vi "_test_BC_FromScratch.vi"() -> ()   [LabVIEW 2020]
uses:
  Source/Libraries/Ballard_1553_Hardware_ni/_typedefs/MessageBuffer_type.ctl
  Source/Libraries/Ballard_1553_Hardware_ni/_typedefs/MessageCommand_BCRT_type.ctl
  <vilib>/addons/_JKI Toolkits/Caraya/classes/Assert/Assert Not Error.vi
  <vilib>/addons/_JKI Toolkits/Caraya/classes/Assert/Assert.lvclass
  <vilib>/addons/_JKI Toolkits/Caraya/classes/Test/Test.lvclass
  Source/Libraries/Ballard_1553_Hardware_ni/Ballard_1553_Hardware_ni.lvlib
panel:
  in  "bus monitor":string="busMonitor"
  in  "major frame":string="testMajorFrame"
  in  "minor frame":string="testMinorFrame"
  in  "message command name":string="testBCmsg"
  in  "message buffer name":string="testBCmsgBuffer"
  in  "BC name":string="testBC"
  in  "channel name":string="channel1553"
  in  "Message Command Configuration":T1={"taVal1"=1, "saVal1"=2, "wordCount1"=1}
  in  "MessageBuffer configuration":T2={"bufferMaxEntries"=1, "bufferType"=0, "eventLogOnEmptyOrFull"=FALSE, "eventLogOnHalf"=FALSE} {"bufferType" items=["FIFO", "Circular"]}
  in  "XML Configuration File Path":path=path "C:/Users/Administrator/Desktop/GIT/Ballard-Arinc-429-XML-Generator/Database Examples/HardwareBallard_1553_Scripted.xml"
  out "error out":errorcluster
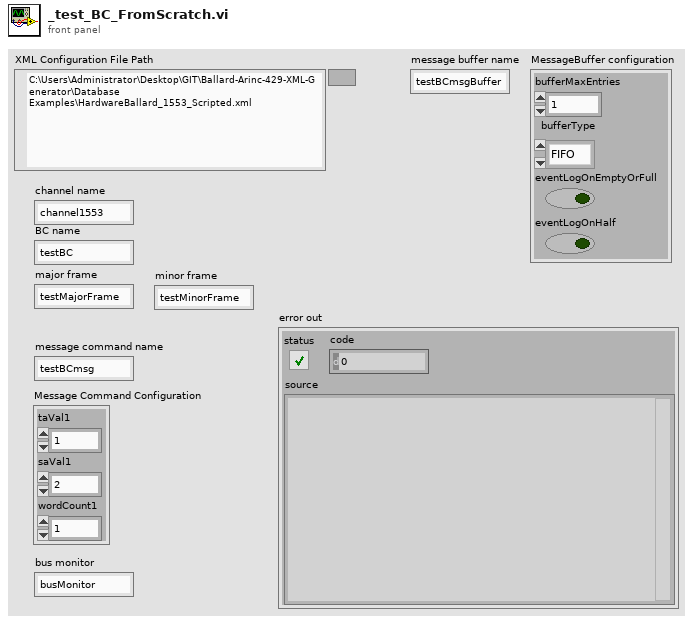
[diagram p1: front panel]
types:
  T1 = typedef "Ballard_1553_Hardware_ni.lvlib/MessageCommand_BCRT_type.ctl" = cluster{"taVal1":i8, "saVal1":i8, "wordCount1":i8}
  T2 = typedef "Ballard_1553_Hardware_ni.lvlib/MessageBuffer_type.ctl" = cluster{"bufferMaxEntries":i32, "bufferType":i32, "eventLogOnEmptyOrFull":bool, "eventLogOnHalf":bool}
  T3 = typedef "Ballard_1553_Hardware_ni.lvlib/schedItem1553_type.ctl" = cluster{"type":T4, "messageIDRef":i32, "singleShot (F)":bool, "skip (F)":bool, "gapTime":dbl}
  T4 = typedef "Ballard_1553_Hardware_ni.lvlib/frame_entry_type.ctl" = enum16{"Message", "Gap", "Pulse", "Log", "Pause", "Restart", "Halt"}
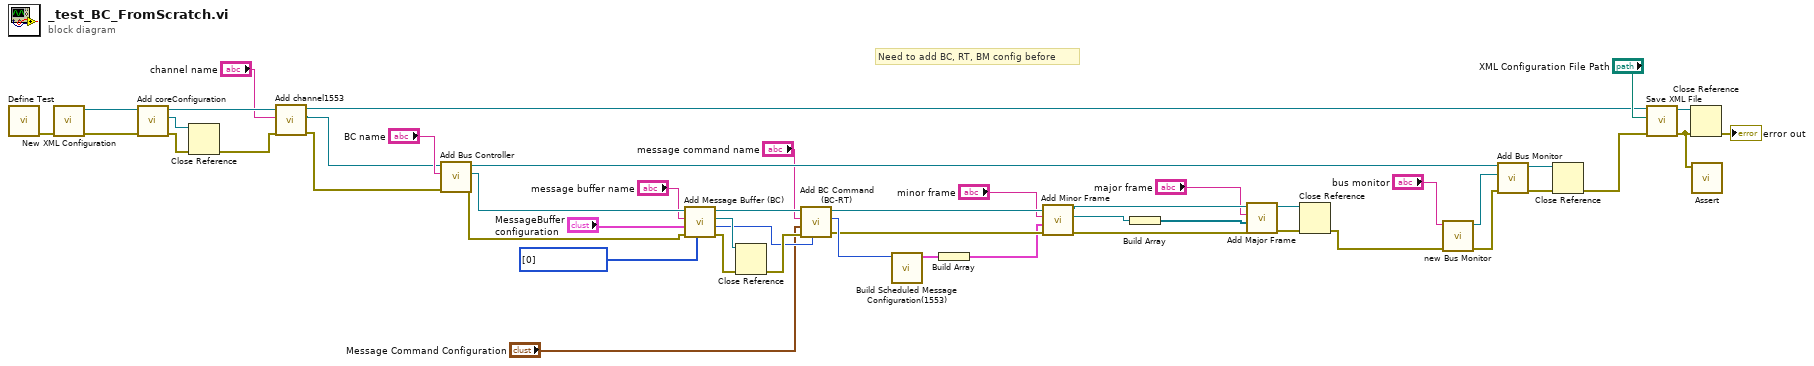
[diagram p0: block diagram]
diagram:
  # "Need to add BC, RT, BM config before"
  n1 = call <vilib>:"Define Test.vi"() -> ("error out"=w9:errorcluster)  [unwired: 11 in]
  n2 = call "New XML Configuration.vi"("error in"=w9) -> ("error out"=w10:errorcluster, "xml ref out"=w11:refnum<k24>)  [unwired: 9 in]
  n3 = call "Add coreConfiguration.vi"("error in"=w10, "xml ref in"=w11) -> ("error out"=w36:errorcluster, "new coreConfiguration out"=w37:refnum<k24>, "xml ref out"=w8:refnum<k24>)  [unwired: 7 in]
  n4 = Close Reference(reference=w37, error in (no error)=w36) -> (error out=w6:errorcluster)
  n5 = call "Add channel1553.vi"("error in"=w6, "name"="channel name", "xml ref in"=w8) -> ("error out"=w5:errorcluster, "new channel1553 out"=w4:refnum<k24>, "xml ref out"=w3:refnum<k24>)  [unwired: 6 in]
  n6 = call "Add Bus Controller.vi"("error in"=w5, "name"="BC name", "1553channel ref in"=w4) -> ("error out"=w24:errorcluster, "new busController"=w31:refnum<k24>, "1553channel ref out"=w45:refnum<k24>)  [unwired: 6 in]
  n7 = call "Add Message Buffer (BC).vi"("MessageData (0x0000)"=u16[] [0], "error in"=w24, "MessageBuffer configuration"="MessageBuffer configuration", "name"="message buffer name", "Bus Controllerl in"=w31) -> ("error out"=w22:errorcluster, "ID out"=w19:i32, "new messageBuffer"=w20:refnum<k24>, "Bus Controller out"=w40:refnum<k24>)  [unwired: 3 in]
  n8 = Close Reference(reference=w20, error in (no error)=w22) -> (error out=w21:errorcluster)
  n9 = call "Add BC Command (BC-RT).vi"("messageBufferIDRef(-1)"=w19, "error in"=w21, "Message Command Configuration"="Message Command Configuration", "name"="message command name", "BusController in"=w40) -> ("error out"=w18:errorcluster, "Message Command ID out"=w27:i32, "BusController out"=w39:refnum<k24>)  [unwired: 4 in]
  n10 = call "Build Scheduled Message Configuration(1553).vi"("messageIDRef"=w27) -> ("1553 Scheduled Message Configuration out"=w38:T3)  [unwired: 10 in]
  n11 = Build Array(w38) -> (w17:T3[])
  n12 = call "Add Minor Frame.vi"("error in"=w18, "Scheduled Message Config in"=w17, "name"="minor frame", "BusController in"=w39) -> ("error out"=w15:errorcluster, "new Minor Frame"=w12:refnum<k24>, "BusController out"=w41:refnum<k24>)  [unwired: 5 in]
  n13 = Build Array(w12) -> (w13:refnum<k24>[])
  n14 = call "Add Major Frame.vi"("error in"=w15, "Minor Frames"=w13, "name"="major frame", "BusController in"=w41) -> ("error out"=w29:errorcluster, "BusController out"=w28:refnum<k24>)  [unwired: 6 in]
  n15 = Close Reference(reference=w28, error in (no error)=w29) -> (error out=w30:errorcluster)
  n16 = call "new Bus Monitor.vi"("error in"=w30, "name"="bus monitor") -> ("error out"=w44:errorcluster, "busMonitor out"=w42:refnum<k24>)  [unwired: 8 in]
  n17 = call "Add Bus Monitor.vi"("error in"=w44, "new busMonitor"=w42, "1553channel ref in"=w45) -> ("error out"=w35:errorcluster, "1553channel ref out"=w33:refnum<k24>)  [unwired: 7 in]
  n18 = Close Reference(reference=w33, error in (no error)=w35) -> (error out=w34:errorcluster)
  n19 = call "Save XML File.vi"("error in"=w34, "XML Configuration File Path"="XML Configuration File Path", "xml ref in"=w3) -> ("error out"=w47:errorcluster, "xml ref out"=w48:refnum<k24>)  [unwired: 7 in]
  n20 = Close Reference(reference=w48, error in (no error)=w47) -> (error out=→"error out":errorcluster)
  n21 = call-poly <vilib>:"Assert.vi"("Not Error?"=w47) -> ()  [unwired: 10 in, 1 out]
